vi "p21forArduino.vi"() -> ()   [LabVIEW 2023]
uses:
  <vilib>/MakerHub/LINX/Public/Peripherals/PWM/PWM Set Duty Cycle 1 Chan.vi
  <vilib>/MakerHub/LINX/Public/Peripherals/Analog/Analog Read 1 Chan.vi
  <vilib>/MakerHub/LINX/Public/Peripherals/Analog/Analog Read N Chans.vi
  <vilib>/MakerHub/LINX/Private/Local IO/LinxAnalogRead.vi
  <vilib>/MakerHub/LINX/Public/Utilities/Check Channel.vi
  <vilib>/MakerHub/LINX/Public/Utilities/Open Serial.vi
  <vilib>/MakerHub/LINX/Public/Peripherals/PWM/PWM Set Duty Cycle N Chans.vi
  <vilib>/MakerHub/LINX/Private/Utilties/Generate Error.vi
  <vilib>/MakerHub/LINX/LMH-LINX.lvlib
panel:
  in  "amplitud":dbl
  out "Waveform Chart 2":dynamicdata(graph)
  in  "PWM Channel":u8
  in  "analog control":u8
  out "Error Out, created indicator":errorcluster
  out "Waveform Chart":dbl(graph)
  in  "t0":dbl
  in  "tsim":dbl
  out "T":dbl
  out "ns":dbl
  in  "fs muestreo":dbl
  # "si no les das valores a los input la onda no se muestra, se cancela, pueden ocurrir errores"
  # "we are gonna make the formula ts/T + 1"
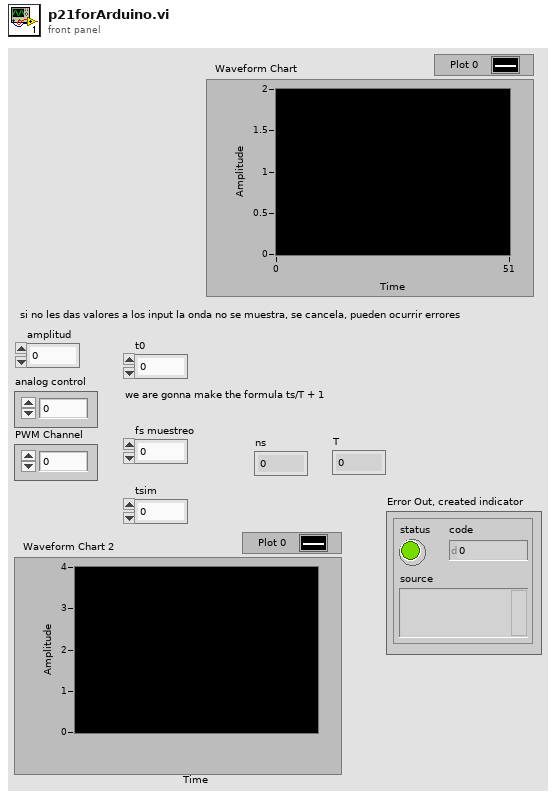
[diagram p1: front panel]
types:
  T1 = typedef "LMH-LINX.lvlib/LINX Ref.ctl" = cluster{"IO":T2, "Interface":T3, "LINX Device Config":T4}
  T2 = typedef "LMH-LINX.lvlib/Platform.ctl" = enum16{"Remote", "Local"}
  T3 = typedef "LMH-LINX.lvlib/Interface.ctl" = enum16{"Serial", "TCP"}
  T4 = typedef "LMH-LINX.lvlib/Device.lvlib/LINX Device Config.ctl" = cluster{"Interface":T3, "COM Port":refnum<visa-resource-name>, "TCP Configuration":T5, "Device Family":u8, "Device ID":u8, "Device Name":string, "TCP Ref":refnum<k5>, "Channels":T6}
  T5 = typedef "LMH-LINX.lvlib/Device.lvlib/TCP Config.ctl" = cluster{"IP Address":string, "Port":u16}
  T6 = typedef "LMH-LINX.lvlib/Channels.ctl" = cluster{"DI":u8[], "DO":u8[], "AI":u8[], "AO":u8[], "PWM":u8[], "QE":u8[], "UART":u8[], "I2C 2":u8[], "SPI":u8[], "CAN":u8[], "Servo":u8[], "AI Ref (V)":dbl, "AI Resolution (Bits)":u8, "AO Ref (V)":dbl, "AO Resolution (Bits)":u8}
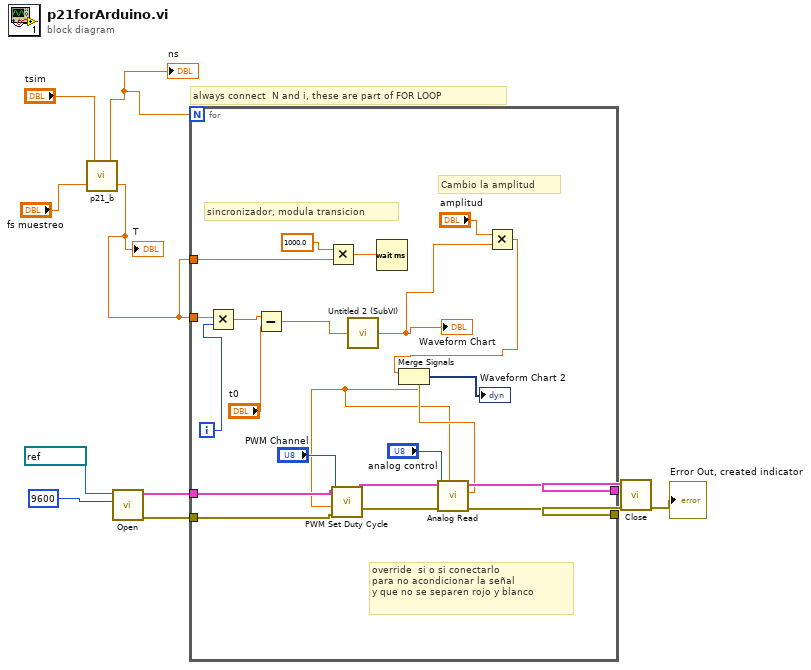
[diagram p0: block diagram]
diagram:
  # "always connect  N and i, these are part of FOR LOOP"
  n1 = call "p21_b.vi"("fs muestreo"="fs muestreo", "tsim"="tsim") -> ("T"=w9:dbl, "NS"=w8:dbl)
  "ns" <- w8
  "T" <- w9
  n2 = call-poly <vilib>:"Open.vi"("Baud Rate Override"=u32 9600, "Serial Port"=refnum<visa-resource-name> "COM7") -> ("Error Out"=w5:errorcluster, "LINX Resource"=w7:T1)  [unwired: 7 in, 1 out]
  n3 = for {
    N: w8 -> [_]
    tunnel: w9 -> [w27]
    tunnel: w9 -> [w25]
    tunnel: w7 -> [w24]
    tunnel: [w20] -> w6
    tunnel: w5 -> [w23]
    tunnel: [w19] -> w4
    i -> [w26]
    # "override  si o si conectarlo\npara no acondicionar la señal \ny que no se separen rojo y blanco"
    # "Cambio la amplitud"
    # "sincronizador, modula transicion"
    n4 = Multiply(x=w27, y=w26) -> (x*y=w30:dbl)
    n5 = Subtract(x=w30, y="t0") -> (x-y=w28:dbl)
    n6 = Multiply(x=1000.0, y=w25) -> (x*y=w31:dbl)
    n7 = call "Untitled 2 (SubVI).vi"("input"=w28) -> ("output"=w13:dbl)
    "Waveform Chart" <- w13
    n8 = Wait (ms)(milliseconds to wait=w31) -> ()  [unwired: 1 out]
    n9 = Multiply(x="amplitud", y=w13) -> (x*y=w12:dbl)
    n10 = call-poly <vilib>:"PWM Set Duty Cycle.vi"("Error In"=w23, "Duty Cycle (0-1)"=w12, "PWM Channel"="PWM Channel", "LINX Resource"=w24) -> ("Error Out"=w21:errorcluster, "LINX Resource"=w22:T1)  [unwired: 6 in]
    n11 = call-poly <vilib>:"Analog Read.vi"("Analog Ref Override (V)"=w12, "Error In"=w21, "Analog Channel"="analog control", "LINX Resource"=w22) -> ("Error Out"=w19:errorcluster, "Voltage"=w16:dbl, "LINX Resource"=w20:T1)  [unwired: 4 in, 1 out]
    n12 = Merge Signals(w12, w16) -> (→"Waveform Chart 2":dynamicdata)
  }
  n13 = call <vilib>:"Close.vi"("Error In"=w4, "LINX Resource"=w6) -> ("Error Out"=→"Error Out, created indicator":errorcluster)  [unwired: 9 in]
